vi "SetTemperature.vi"(8 "error in (no error)":errorcluster, 10 "TSetpoint(degC/100)":i16, 11 "CameraSession  in":refnum<class "CS250-CameraHardwareClass.lvclass">) -> (0 "error out":errorcluster, 1 "Success":bool, 2 "TSetpointReadback(degC/100)":i16, 3 "CameraSession out":refnum<class "CS250-CameraHardwareClass.lvclass">)   [LabVIEW 2013, in "CS250-CameraHardwareClass.lvclass"]
uses:
  CS250-CameraHardwareClass.lvclass
  CS250-CameraHardwareClass.lvclass/CS250-CameraHardwareClass.ctl
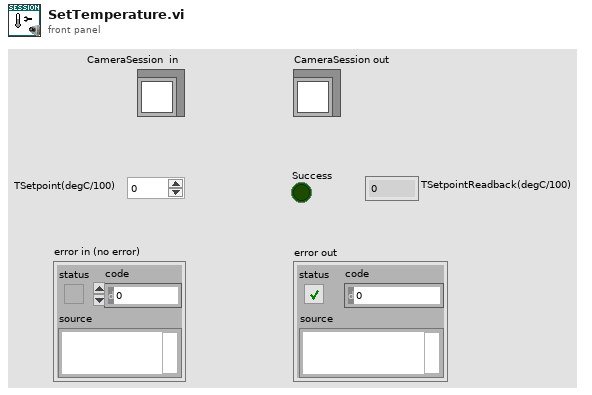
[diagram p1: front panel]
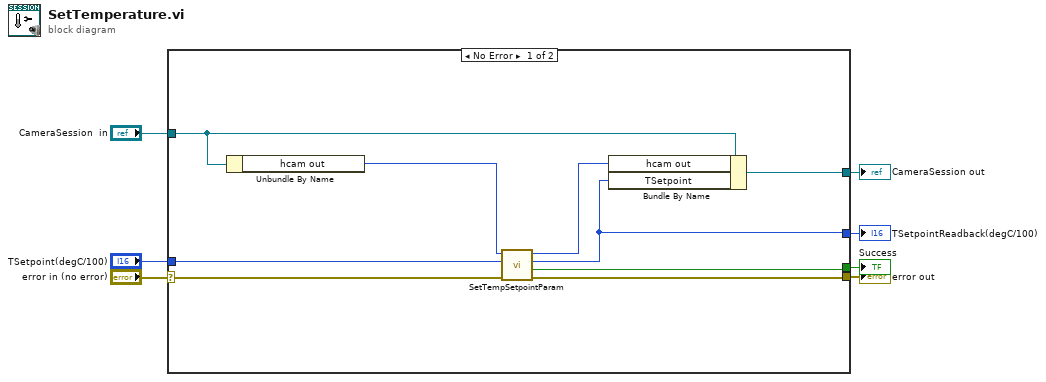
[diagram p0: block diagram]
diagram:
  n1 = case shown="No Error" "error in (no error)" {
    selector: "error in (no error)" -> [w15 w17]
    tunnel: [w10 w18] -> w6
    tunnel: "CameraSession  in" -> [w16 w18]
    tunnel: [w14 w17] -> w4
    tunnel: [w12 _] -> w3
    tunnel: "TSetpoint(degC/100)" -> [w9 _]
    tunnel: [w8 _] -> w1
    frame No Error {
      n2 = Unbundle By Name(w16) -> ("hcam out"=w13:i16)
      n3 = call "SetTempSetpointParam.vi"("error in (no error)"=w15, "TSetpoint(degC/100)"=w9, "hcam in"=w13) -> ("error out"=w14:errorcluster, "Success"=w12:bool, "TSetpointReadback(degC/100)"=w8:i16, "hcam out"=w11:i16)  [unwired: 5 in]
      n4 = Bundle By Name(cluster=w16, "hcam out"=w11, "TSetpoint"=w8) -> (w10:refnum<class "CS250-CameraHardwareClass.lvclass">)
    }
    frame Error {
    }
  }
  "CameraSession out" <- w6
  "Success" <- w3
  "error out" <- w4
  "TSetpointReadback(degC/100)" <- w1
